vi "15 Messing with Time.vi"() -> ()   [LabVIEW 2019]
uses:
  _Subs/OpenDiagram/Open_XControl.xctl
panel:
  out "year":i32
  out "string of info":string
  out "Cluster of Info":T1
  out "seconds different":dbl
  in  "Set time":timestamp=timestamp(3650374200 s since 1904-01-01)
  out "current time":timestamp
  in  "OpenDiag":refnum<vi>(xcontrol)
  # "15 Messing with Time\nThis code shows some examples of how to use LabVIEW time\n\nInstructions:\n1. Hit Run, look at all the ways of extracting time information\n2. Change the Set time and run again (click on calendar icon)"
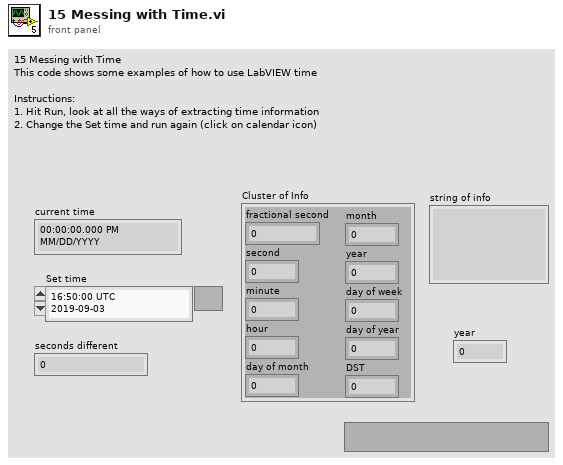
[diagram p1: front panel]
types:
  T1 = cluster{"fractional second":dbl, "second":i32, "minute":i32, "hour":i32, "day of month":i32, "month":i32, "year":i32, "day of week":i32, "day of year":i32, "DST":i32}
  T2 = typedef "LVDateTimeRec.ctl" = cluster{"fractional second":dbl, "second":i32, "minute":i32, "hour":i32, "day of month":i32, "month":i32, "year":i32, "day of week":i32, "day of year":i32, "DST":i32}
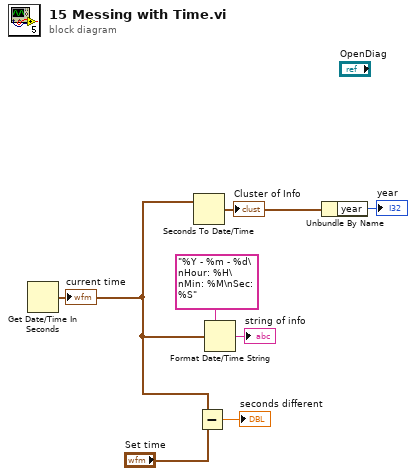
[diagram p0: block diagram]
diagram:
  n1 = Get Date/Time In Seconds() -> (seconds since 1Jan1904=w3:timestamp)
  "current time" <- w3
  n2 = Seconds To Date/Time(time stamp (now)=w3) -> (date time rec=w2:T2)  [unwired: 1 in]
  "Cluster of Info" <- w2
  n3 = Subtract(x=w3, y="Set time") -> (x-y=→"seconds different":dbl)
  n4 = Format Date/Time String(time format string (%c)="%Y - %m - %d\nHour: %H\nMin: %M\nSec: %S", seconds (now)=w3) -> (date/time string=→"string of info":string)  [unwired: 1 in]
  n5 = Unbundle By Name(w2) -> ("year"=→"year":i32)
